vi "Close Logger.vi"(8 "error in":errorcluster) -> (0 "error out":errorcluster, 3 "Error Logger out":refnum<class "Error Logger.lvclass">)   [LabVIEW 2012, in "Error Logger.lvclass"]
uses:
  Error Logger.lvclass
  Error Logger.lvclass/Error Logger.ctl
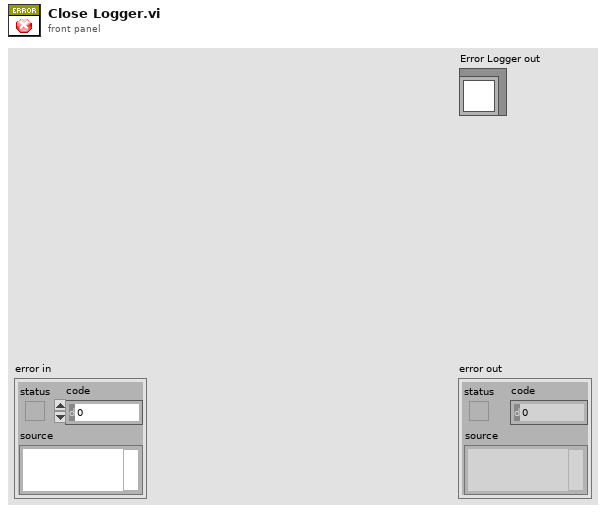
[diagram p1: front panel]
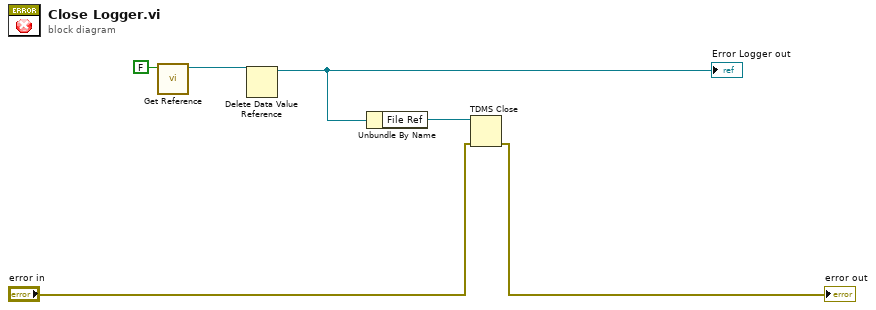
[diagram p0: block diagram]
diagram:
  n1 = call "Get Reference.vi"("Init?"=FALSE) -> ("DVR"=w5:refnum<data-value>)  [unwired: 9 in, 1 out]
  n2 = Delete Data Value Reference(data value reference=w5) -> (data value=w4:refnum<class "Error Logger.lvclass">)  [unwired: 1 in, 1 out]
  "Error Logger out" <- w4
  n3 = Unbundle By Name(w4) -> ("File Ref"=w3:refnum<k34>)
  n4 = TDMS Close(8:"error in", 11:w3) -> (0:→"error out":errorcluster)  [unwired: 1 out]
